vi "Signal Timer.vi"(0 "Input":bool, 1 "Edge":bool, 2 "Interval":dbl format="%#_13g", 3 "Pull":bool=TRUE) -> (4 "Filtered Output":bool)   [LabVIEW 2016]
uses:
  Change Detect Boolean.vi
panel:
  # "Signal"
  # "Pulled Up"
  # "on DOWN edge"
  # "Pulled Down"
  # "on UP edge"
  # "?"
  # "?"
  # "?"
  # "?"
  # "?"
  # "?"
  # "?"
  # "?"
  # "Intervals influenced by Timer\n(of specified length, in ms)"
  # "Invervals immediately after T/F transitions can be pulled either UP or DOWN"
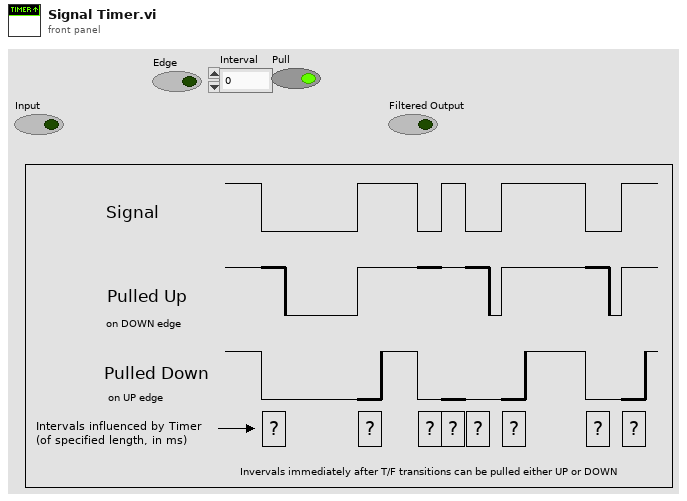
[diagram p1: front panel]
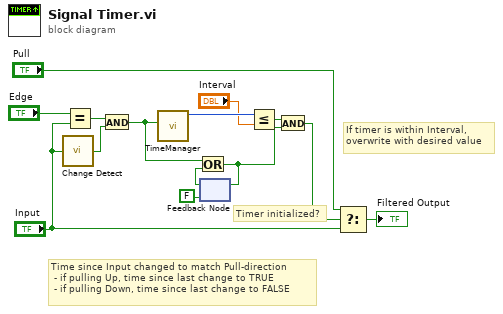
[diagram p0: block diagram]
diagram:
  # "Timer initialized?"
  # "If timer is within Interval,\noverwrite with desired value"
  # "Time since Input changed to match Pull-direction\n - if pulling Up, time since last change to TRUE\n - if pulling Down, time since last change to FALSE"
  n1 = call-poly "Change Detect.vi"("In"="Input") -> ("Changed?"=w3:bool)
  n2 = Equal?(x="Edge", y="Input") -> (x = y?=w2:bool)
  n3 = And(x=w2, y=w3) -> (x .and. y?=w4:bool)
  n4 = call "TimeManager.vi"("Reset?"=w4) -> ("Time Since Reset"=w14:u32)  [unwired: 9 in, 1 out]
  n5 = feedback #1(FALSE ("Input")) -> (w9:bool)
  n6 = Or(x=w4, y=w9) -> (x .or. y?=w6:bool)
  n7 = feedback-in #1(w6) -> ()
  n8 = Less Or Equal?(x=w14, y="Interval") -> (x <= y?=w8:bool)
  n9 = And(x=w8, y=w6) -> (x .and. y?=w7:bool)
  n10 = Select(t="Pull", s=w7, f="Input") -> (s? t:f=→"Filtered Output":bool)
